vi "Scale Color.vi"(4 "Brightness":u8, 6 "Factor":dbl, 9 "Red":u8, 10 "Green":u8, 11 "Blue":u8) -> (1 "Red Out":u8, 2 "Green Out":u8, 3 "Blue Out":u8)   [LabVIEW 2013]
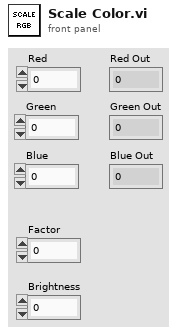
[diagram p1: front panel]
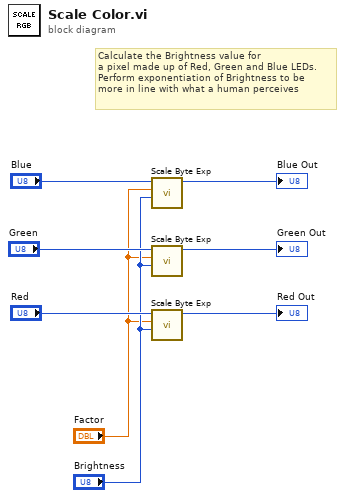
[diagram p0: block diagram]
diagram:
  # "Calculate the Brightness value for\na pixel made up of Red, Green and Blue LEDs.\nPerform exponentiation of Brightness to be\nmore in line with what a human perceives"
  n1 = call "Scale Byte Exp.vi"("Brightness"="Brightness", "Factor"="Factor", "Byte"="Blue") -> ("Byte Scaled"=→"Blue Out":u8)  [unwired: 8 in]
  n2 = call "Scale Byte Exp.vi"("Brightness"="Brightness", "Factor"="Factor", "Byte"="Green") -> ("Byte Scaled"=→"Green Out":u8)  [unwired: 8 in]
  n3 = call "Scale Byte Exp.vi"("Brightness"="Brightness", "Factor"="Factor", "Byte"="Red") -> ("Byte Scaled"=→"Red Out":u8)  [unwired: 8 in]
